vi "GLdrv_DATA_CAPT.vi"(0 "Connection ID":T1, 5 "Capture":enum16{"DISK"}(ring), 7 "File":string, 11 "error in (no error)":errorcluster, 13 "Query(f)":bool) -> (4 "Connection ID Out":T1, 6 "Capture out":enum16{"DISK"}(ring), 8 "File out":string, 15 "error out":errorcluster)   [LabVIEW 2017, in "GL860_Driver.lvlib"]
doc: "データの収録先の設定・参照\nDISK=MEM/SD\n例)MEM: DATA:CAPT DISK,”\\MEM\\FOLDER\\0001.GBD”\n例)自動ファイル名にする時: DATA:CAPT DISK,\"\\MEMs\\FOLDER\\”\n　（パスにフォルダを指定した場合は自動ファイル名となり、そのフォル\nダに日付-時刻のフォルダが作成され、データは日付-時刻のフォルダ\nの中に保存されます。)"
uses:
  GL860_Driver.lvlib
  ConnectionID.ctl
  GLdrv_RW.ctl
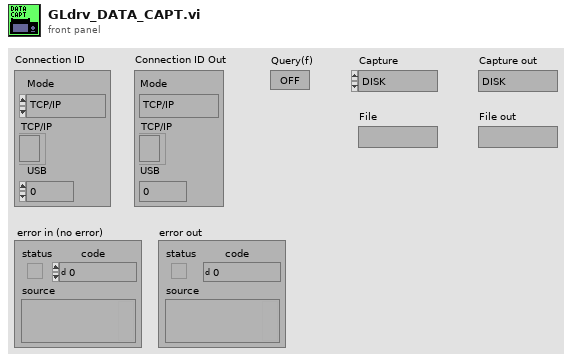
[diagram p1: front panel]
types:
  T1 = typedef "ConnectionID.ctl" = cluster{"Mode":enum16{"TCP/IP", "USB"}, "TCP/IP":refnum<k5>, "USB":i32}
  T2 = typedef "GLdrv_RW.ctl" = enum16{"Auto", "Read", "Write", "Buffer"}
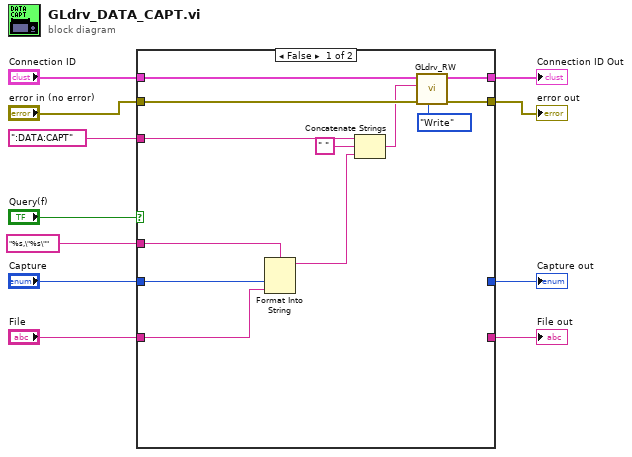
[diagram p0: block diagram]
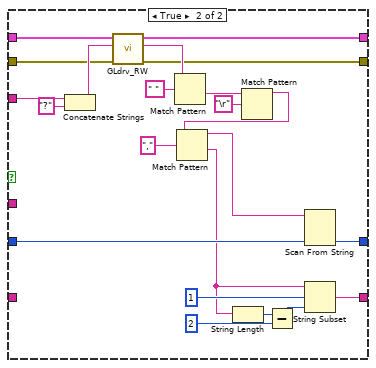
[diagram p2: hidden frame]
diagram:
  n1 = case shown="FALSE" "Query(f)" {
    tunnel: ":DATA:CAPT" ("Command") -> [w23 w42]
    tunnel: [w18 w35] -> w11
    tunnel: [w20 w39] -> w10
    tunnel: "Connection ID" -> [w21 w40]
    tunnel: "error in (no error)" -> [w19 w36]
    tunnel: "Capture" -> [w12 w34]
    tunnel: [_ w33] -> w3
    tunnel: "%s,\"%s\"" ("Param") -> [w14 _]
    tunnel: [_ w24] -> w2
    tunnel: "File" -> [w13 _]
    frame False {
      n2 = Format Into String(format string=w14, w12, w13) -> (resulting string=w15:string)  [unwired: 2 in, 1 out]
      n3 = Concatenate Strings(w23, " " ("string"), w15) -> (w17:string)
      n4 = call "GLdrv_RW.vi"("Mode(read)"=GLdrv_RW."Write", "error in (no error)"=w19, "data in"=w17, "Connection ID"=w21) -> ("error out"=w18:errorcluster, "Connection ID Out"=w20:T1)  [unwired: 3 in, 3 out]
    }
    frame True {
      n5 = Concatenate Strings(w42, "?" ("string")) -> (w38:string)
      n6 = call "GLdrv_RW.vi"("error in (no error)"=w36, "data in"=w38, "Connection ID"=w40) -> ("error out"=w35:errorcluster, "data out"=w37:string, "Connection ID Out"=w39:T1)  [unwired: 4 in, 2 out]
      n7 = Match Pattern(string=w37, regular expression=" " ("search string/char (-)")) -> (after substring=w43:string)  [unwired: 4 out]
      n8 = Match Pattern(string=w43, regular expression="\r") -> (before substring=w30:string)  [unwired: 4 out]
      n9 = Match Pattern(string=w30, regular expression=",") -> (before substring=w31:string, after substring=w25:string)  [unwired: 3 out]
      n10 = String Length(string=w25) -> (length=w28:i32)
      n11 = Subtract(x=w28, y=2) -> (x-y=w27:i32)
      n12 = Scan From String(input string=w31, default 1=w34) -> (output 1=w33:enum16{"DISK"})  [unwired: 3 in, 3 out]
      n13 = String Subset(string=w25, offset (0)=1, length (rest)=w27) -> (substring=w24:string)
    }
  }
  "Connection ID Out" <- w10
  "error out" <- w11
  "Capture out" <- w3
  "File out" <- w2
